vi "List.vi"(8 "error in (no error)":errorcluster) -> (0 "error out":errorcluster, 3 "All Timers":T1(array[cluster]))   [LabVIEW 2018, in "QueueTimer.lvlib"]
doc: "List all queue timers in memory. This groups the queue timers by queue reference."
uses:
  QueueTimer.lvlib
  <vilib>/Utility/miscctls.llb/LVMapReplaceAction.ctl
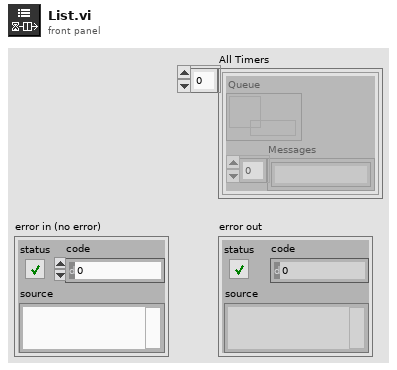
[diagram p1: front panel]
types:
  T1 = cluster{"Queue":refnum<queue>, "Messages":string[]}[]
  T2 = typedef "LVMapReplaceAction.ctl" = enum32{"Modify Entry only if found", "Add or Modify Entry", "Delete Entry"}
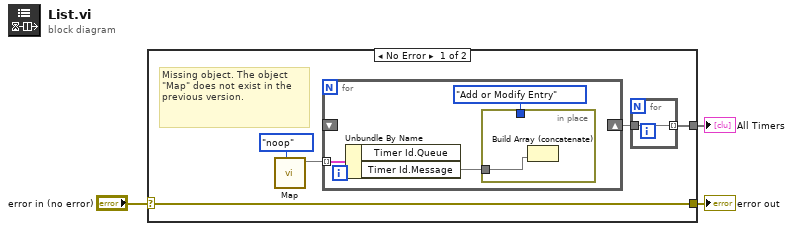
[diagram p0: block diagram]
diagram:
  # "Missing object. The object \"Map\" does not exist in the previous version."
  n1 = case shown="No Error" "error in (no error)" {
    selector: "error in (no error)" -> [w4 w17]
    tunnel: [w5 _] -> w3
    tunnel: [w4 w17] -> w2
    frame No Error {
      n2 = call "Map.vi"("Action"=enum8{"noop", "get", "set", "pop"}."noop") -> (3:w8)  [unwired: 8 in, 2 out]
      n3 = for {
        tunnel: w8 -> [w14] mode=indexing
        shift-right: [_] -> w6
        shift-left: [w13] -> w7
        n4 = Unbundle By Name(w14) -> ("Timer Id.Queue"=w11, "Timer Id.Message"=w10)
        n5 = in-place {
          in-place-border: LVMapReplaceAction."Add or Modify Entry" ("action") -> [_]
          in-place-border: w10 -> [w15]
          n6 = Build Array (concatenate)(w15) -> ()  [unwired: 1 in, 1 out]
        }
      }
      n7 = for {
        tunnel: w6 -> [w16]
        tunnel: [w16] -> w5 mode=indexing
      }
    }
    frame Error {
    }
  }
  "error out" <- w2
  "All Timers" <- w3
